vi "LVRT Serial Write.vi"(8 "error in (no error)":errorcluster, 10 "String":string="*IDN?\n", 11 "FPGA Main Ref":T1) -> (0 "error out":errorcluster, 3 "FPGA Main Ref Out":T1)   [LabVIEW 2009]
uses:
  serial FPGA main reference type def.ctl
  <vilib>/rvi/interface/nirviReadWriteControl/nirviReadWriteControl.xnode
  FPGA Bitfiles/Athena Brain.lvproj_FPGA Target 2_serial FPGA Main.vi.lvbitx
  serial FPGA Main.vi
  <vilib>/Utility/error.llb/Error Cluster From Error Code.vi
  <vilib>/rvi/errors/niLvFpgaAdjustHostInterfaceError.vi
  <vilib>/rvi/interface/common/niFpgaNodeNameForErrorReporting.ctl
  <vilib>/rvi/errors/niLvFpgaWhatHappensToTopLevelVI.ctl
  NiRioSrv.dll
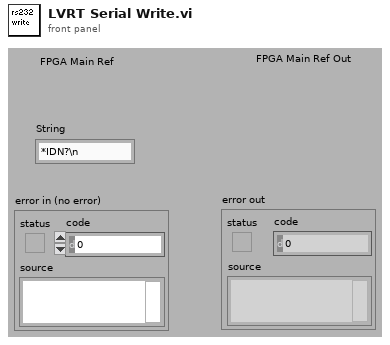
[diagram p1: front panel]
types:
  T1 = typedef "serial FPGA main reference type def.ctl" = refnum<k20>
  T2 = typedef "niFpgaNodeNameForErrorReporting.ctl" = enum16{"Open FPGA VI Reference", "Read/Write Control", "Invoke Method: Abort", "Invoke Method: Acknowledge IRQ", "Invoke Method: Download", "Invoke Method: FIFO.Configure", "Invoke Method: FIFO.Read", "Invoke Method: FIFO.Start", "Invoke Method: FIFO.Stop", "Invoke Method: FIFO.Write", "Invoke Method: Reset", "Invoke Method: Run", "Invoke Method: Wait on IRQ", "Close FPGA VI Reference"}
  T3 = typedef "niLvFpgaWhatHappensToTopLevelVI.ctl" = enum16{"top level VI scripted behind XNode", "top level VI inlined behind XNode"}
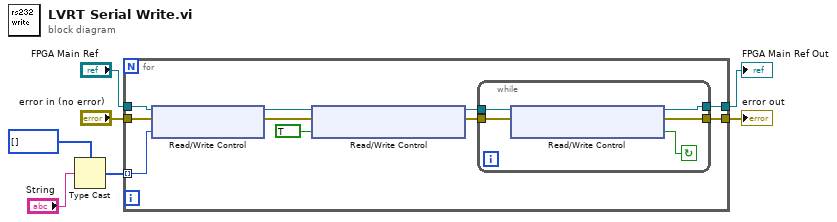
[diagram p0: block diagram]
diagram:
  n1 = Type Cast(type=u8[] [], x="String") -> (*(type *) &x=w4:u8[])
  n2 = for {
    tunnel: "FPGA Main Ref" -> [w14]
    tunnel: [w9] -> w2
    tunnel: "error in (no error)" -> [w13]
    tunnel: [w8] -> w1
    tunnel: w4 -> [w15] mode=indexing
    n3 = xnode "Read/Write Control"("FPGA VI Reference In"=w14, "error in"=w13, "LIDAR Write: Char"=w15) -> ("FPGA VI Reference Out"=w17:T1, "error out"=w16:errorcluster)
    n4 = xnode "Read/Write Control"("FPGA VI Reference In"=w17, "error in"=w16, "LIDAR Write: Data Written"=TRUE ("Data Read")) -> ("FPGA VI Reference Out"=w11:T1, "error out"=w10:errorcluster)
    n5 = while {
      tunnel: w11 -> [w95]
      tunnel: w10 -> [w94]
      tunnel: [w93] -> w9
      tunnel: [w92] -> w8
      stop <- w91 continue-if-true
      n6 = xnode "Read/Write Control"("FPGA VI Reference In"=w95, "error in"=w94) -> ("FPGA VI Reference Out"=w93:T1, "error out"=w92:errorcluster, "LIDAR Write: Data Written"=w91:bool)
    }
  }
  "error out" <- w1
  "FPGA Main Ref Out" <- w2
